vi "Query the model type of Scanner Box.vi"(0 "VISA resource name":refnum<visa-resource-name>, 5 "error in":errorcluster) -> (14 "VISA resource name out":refnum<visa-resource-name>, 15 "Model Type of 1ST":i32, 16 "Model Type of 2ND":i32, 17 "Model Type of 3RD":i32, 18 "Model Type of 4TH":i32, 19 "error out":errorcluster)   [LabVIEW 2011, in "GPT-9000.lvlib"]
uses:
  <instrlib>/GPT-9000/GPT-9000.lvlib
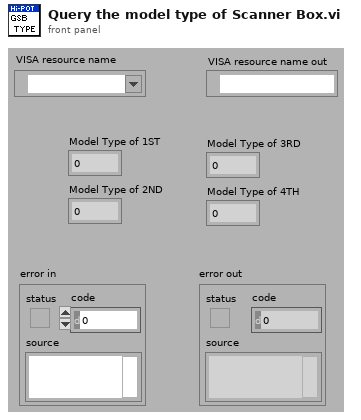
[diagram p1: front panel]
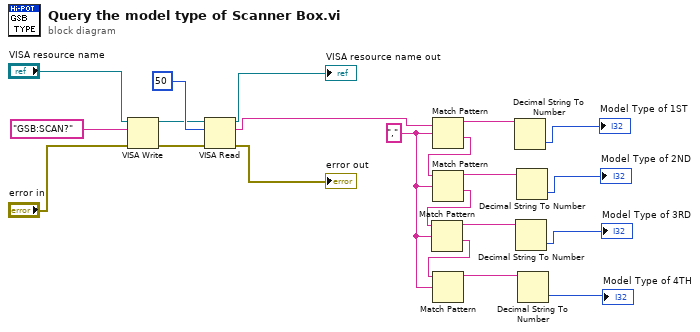
[diagram p0: block diagram]
diagram:
  w9 = "," ("search string/char (-)")
  n1 = VISA Write(VISA resource name="VISA resource name", write buffer="GSB:SCAN?", error in (no error)="error in") -> (VISA resource name out=w17:refnum<visa-resource-name>, error out=w16:errorcluster)  [unwired: 1 out]
  n2 = VISA Read(VISA resource name=w17, byte count=u32 50, error in (no error)=w16) -> (VISA resource name out=→"VISA resource name out":refnum<visa-resource-name>, read buffer=w13:string, error out=→"error out":errorcluster)  [unwired: 1 out]
  n3 = Match Pattern(string=w13, regular expression=w9) -> (before substring=w8:string, after substring=w15:string)  [unwired: 1 in, 2 out]
  n4 = Match Pattern(string=w15, regular expression=w9) -> (before substring=w7:string, after substring=w14:string)  [unwired: 1 in, 2 out]
  n5 = Match Pattern(string=w14, regular expression=w9) -> (before substring=w6:string, after substring=w10:string)  [unwired: 1 in, 2 out]
  n6 = Match Pattern(string=w10, regular expression=w9) -> (before substring=w5:string)  [unwired: 1 in, 3 out]
  n7 = Decimal String To Number(string=w8) -> (number=→"Model Type of 1ST":i32)  [unwired: 2 in, 1 out]
  n8 = Decimal String To Number(string=w6) -> (number=→"Model Type of 3RD":i32)  [unwired: 2 in, 1 out]
  n9 = Decimal String To Number(string=w7) -> (number=→"Model Type of 2ND":i32)  [unwired: 2 in, 1 out]
  n10 = Decimal String To Number(string=w5) -> (number=→"Model Type of 4TH":i32)  [unwired: 2 in, 1 out]
